vi "Queue Is Nested.vi"(10 "Alias":string, 11 "Hello World Queue in":refnum<class "Hello World Queue.lvclass">) -> (2 "Queue Is Nested?":bool)   [LabVIEW 2021, in "Hello World Queue.lvlib" / "Hello World Queue.lvclass"]
uses:
  Hello World Queue.lvclass
  Hello World Queue.lvclass/Hello World Queue.ctl
  jettl/Queue jettl/Queue jettl.lvclass
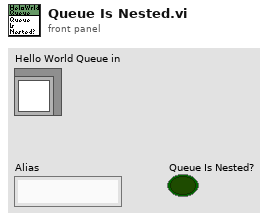
[diagram p1: front panel]
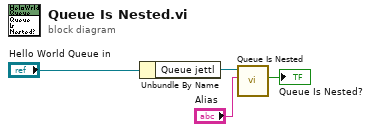
[diagram p0: block diagram]
diagram:
  n1 = Unbundle By Name("Hello World Queue in") -> ("Queue jettl"=w3:refnum<class "Queue jettl.lvclass">)
  n2 = call-dynamic "Queue Is Nested.vi"("Alias"="Alias", "jettl in"=w3) -> ("Queue Is Nested?"=→"Queue Is Nested?":bool)  [unwired: 9 in]
